vi "Radau5_Tolerence Init.vi"(9 "default tolerance":dbl, 10 "width":i32, 11 "Tolerance input":dbl[](array[numeric])) -> (3 "Tolerance output":dbl[](array[numeric]))   [LabVIEW 2020, in "NI_DAE.lvlib"]
uses:
  <vilib>/gmath/NI_DAE.lvlib
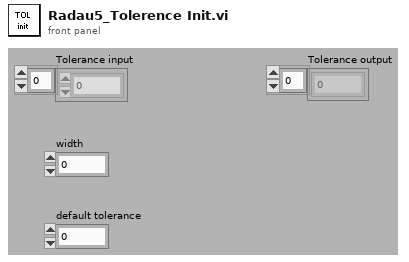
[diagram p1: front panel]
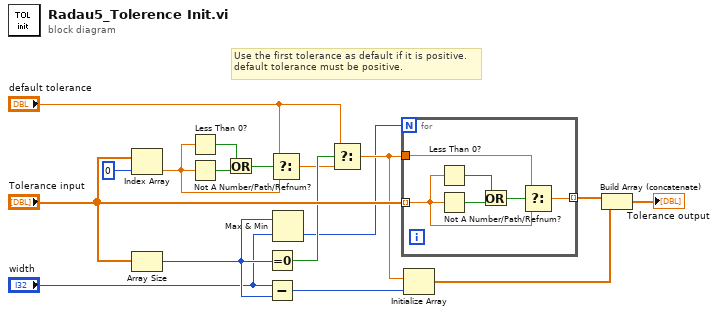
[diagram p0: block diagram]
diagram:
  # "Use the first tolerance as default if it is positive.\ndefault tolerance must be positive."
  n1 = Index Array(array="Tolerance input", index=0) -> (element=w13:dbl)
  n2 = Array Size(array="Tolerance input") -> (size(s)=w3:i32)
  n3 = Less Than 0?(x=w13) -> (x < 0?=w15:bool)
  n4 = Not A Number/Path/Refnum?(number/path/refnum=w13) -> (NaN/Path/Refnum?=w16:bool)
  n5 = Or(x=w15, y=w16) -> (x .or. y?=w14:bool)
  n6 = Equal To 0?(x=w3) -> (x = 0?=w8:bool)
  n7 = Subtract(x="width", y=w3) -> (x-y=w11:i32)
  n8 = Select(t="default tolerance", s=w14, f=w13) -> (s? t:f=w6:dbl)
  n9 = Max & Min(x=w3, y="width") -> (min(x,y)=w1:i32)  [unwired: 1 out]
  n10 = Select(t="default tolerance", s=w8, f=w6) -> (s? t:f=w5:dbl)
  n11 = for {
    N: w1 -> [_]
    tunnel: "Tolerance input" -> [w18] mode=indexing
    tunnel: [w20] -> w10 mode=indexing
    tunnel: w5 -> [w19]
    n12 = Less Than 0?(x=w18) -> (x < 0?=w22:bool)
    n13 = Not A Number/Path/Refnum?(number/path/refnum=w18) -> (NaN/Path/Refnum?=w23:bool)
    n14 = Or(x=w22, y=w23) -> (x .or. y?=w21:bool)
    n15 = Select(t=w19, s=w21, f=w18) -> (s? t:f=w20:dbl)
  }
  n16 = Initialize Array(w5, w11) -> (w9:dbl[])
  n17 = Build Array (concatenate)(w10, w9) -> (→"Tolerance output":dbl[])
